vi "XMLTypeDef_toTimeGrpClass.vi"(8 "error in (no error)":errorcluster, 10 "XML String":string, 11 "TimingGrp":T1) -> (0 "error out":errorcluster, 3 "TimingGrp out":refnum<class "TimingGrp.lvclass">)   [LabVIEW 2018, in "Configuration Grandmaster.lvlib" / "ChassisCfg.lvclass"]
uses:
  ChassisCfg.lvclass
  Class Timing Group/TimingGrp.lvclass
  Custom Ctrls/Master CfgXML/ge_XMLHdr_TimingGrp.ctl
  Custom Ctrls/Master CfgXML/ge_XMLHdr_ChanGroups.ctl
  Custom Ctrls/Master Cfg/ge_GrpHdr.ctl
  Custom Ctrls/ge_MeasType.ctl
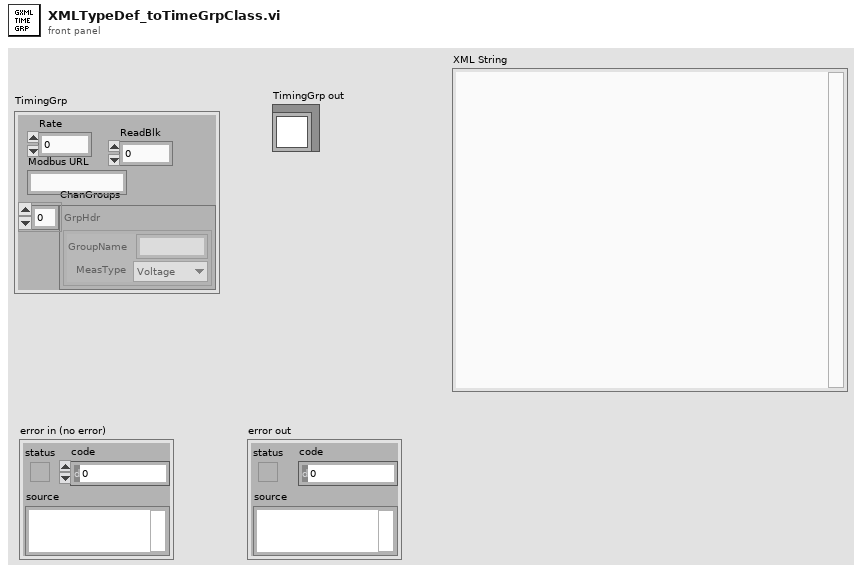
[diagram p1: front panel]
types:
  T1 = typedef "ge_XMLHdr_TimingGrp.ctl" = cluster{"Rate":dbl, "ReadBlk":i32, "Modbus URL":string, "ChanGroups":T2}
  T2 = typedef "ge_XMLHdr_ChanGroups.ctl" = T3[]
  T3 = typedef "ge_GrpHdr.ctl" = cluster{"GroupName":string, "MeasType":T4}
  T4 = typedef "ge_MeasType.ctl" = enum16{"Voltage", "Frequency", "Tachometer", "Dynamic", "Thermocouple", "RTD", "Strain", "Current", "Resistance"}
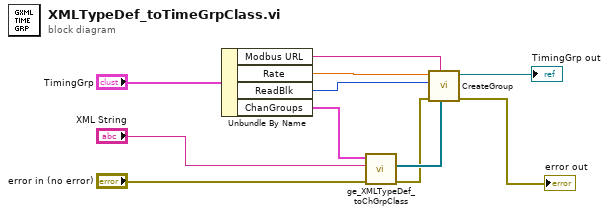
[diagram p0: block diagram]
diagram:
  n1 = Unbundle By Name("TimingGrp") -> ("Modbus URL"=w7:string, "Rate"=w5:dbl, "ReadBlk"=w6:i32, "ChanGroups"=w4:T2)
  n2 = call "ge_XMLTypeDef_toChGrpClass.vi"("error in"="error in (no error)", "GXML String"="XML String", "ChanGroups"=w4) -> ("error out"=w8:errorcluster, "ChanGrp"=w9:refnum<class "ChanGrp.lvclass">[])  [unwired: 7 in]
  n3 = call "CreateGroup.vi"("ChanGroups"=w9, "Modbus URL"=w7, "error in"=w8, "ReadBlk"=w6, "Rate"=w5) -> ("error out"=→"error out":errorcluster, "Timing Group"=→"TimingGrp out":refnum<class "TimingGrp.lvclass">)  [unwired: 5 in]
